vi "Configure Math (Advanced).vi"(7 "Destination (4:Math1)":u16(ring)=4 items=["Math1"=4, "Math2"=5, "Math3"=6, "Math4"=7], 8 "error in (no error)":errorcluster, 10 "Expression":string, 11 "VISA resource name":refnum<visa-resource-name>) -> (0 "error out":errorcluster, 3 "VISA resource name out":refnum<visa-resource-name>)   [LabVIEW 2011, in "Tektronix 7000 Series.lvlib"]
doc: "Configures a math channel using a mathematical expression.You can use Configure Math Expression VI to create a valid math expression or refer to the instrument documenation for syntax of valid math expressions."
uses:
  Tektronix 7000 Series.lvlib
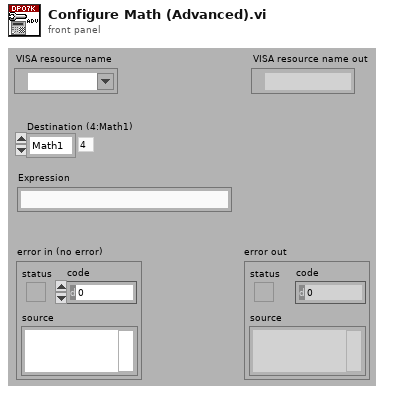
[diagram p1: front panel]
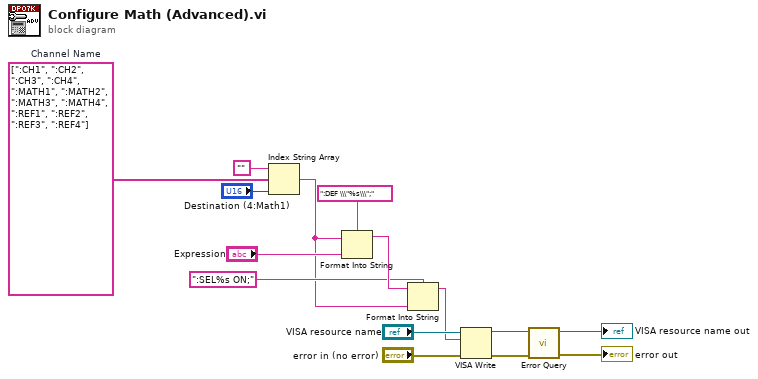
[diagram p0: block diagram]
diagram:
  w15 = string[] [":CH1", ":CH2", ":CH3", ":CH4", ":MATH1", ":MATH2", ":MATH3", ":MATH4", ":REF1", ":REF2", ":REF3", ":REF4"]  # Channel Name
  n1 = Index String Array(1:"Destination (4:Math1)", 2:w15, 3:"") -> (0:w4:string)
  n2 = Format Into String(format string=":DEF \\\"%s\\\";", initial string=w4, "Expression") -> (resulting string=w6:string)  [unwired: 1 in, 1 out]
  n3 = Format Into String(format string=":SEL%s ON;", initial string=w6, w4) -> (resulting string=w3:string)  [unwired: 1 in, 1 out]
  n4 = VISA Write(VISA resource name="VISA resource name", write buffer=w3, error in (no error)="error in (no error)") -> (VISA resource name out=w10:refnum<visa-resource-name>, error out=w9:errorcluster)  [unwired: 1 out]
  n5 = call "Error Query.vi"("error in (no error)"=w9, "VISA resource name"=w10) -> ("error out"=→"error out":errorcluster, "VISA resource name out"=→"VISA resource name out":refnum<visa-resource-name>)  [unwired: 6 in, 2 out]
